vi "Test Broadcast Seen from Process Added After Attaching to Owning Application.vi"(8 "error in (no error)":errorcluster, 11 "Test Case In":refnum<class "Monitor Broadcasts Test.lvclass">) -> (0 "error out":errorcluster, 3 "Test Case Out":refnum<class "Monitor Broadcasts Test.lvclass">)   [LabVIEW 2020, in "Monitor Broadcasts Test.lvclass"]
uses:
  Monitor Broadcasts Test.lvclass
  C:/Program Files (x86)/National Instruments/LabVIEW 2020/vi.lib/Astemes/LUnit/Test Case.lvclass
  source/Broadcast Message Receiver/Broadcast Message Receiver.lvclass
  C:/Git/astemes-triarc-debugger/source/Process/Debug Process.lvclass
  <vilib>/Astemes/Triarc Framework/Application/Application.lvclass
  C:/Program Files (x86)/National Instruments/LabVIEW 2020/vi.lib/Astemes/Triarc Framework/Process/Process.lvclass
  <vilib>/Astemes/Triarc Framework/Process/Process.lvclass
  source/Process/Debug Process.lvclass/Debug Process.ctl
  source/Broadcast Message Receiver/Broadcast Message Receiver.lvclass/Broadcast Message Receiver.ctl
  <vilib>/Astemes/Triarc Framework/Process/Process.lvclass/Process.ctl
  <vilib>/Astemes/Triarc Framework/Application/Application.lvclass/Application.ctl
  <vilib>/Astemes/LUnit/Test Case.lvclass/Test Case.ctl
  b8133177-6539-48d7-afde-5fbce34c741b.vi
  b0973c52-cbc2-441f-a849-3f0b3eb3c153.vi
  01074fa8-ee8a-411d-bc8b-fc92c4f90959.vi
  source/Process/Public/Lifecycle/Get Lifecycle State.vi
  source/Process/Protected/Messaging/Enqueue Message.vi
  <vilib>/Astemes/Triarc Framework/Application/Private/Add Process to Map.vi
  <vilib>/Astemes/Triarc Framework/Application/Private/Throw Error If Process Already in App.vi
  <vilib>/Astemes/Triarc Framework/Process/Protected/Messaging/Send Message.vi
  <vilib>/Astemes/Triarc Framework/Process/Public/Lifecycle/Get Lifecycle State.vi
  <vilib>/Astemes/Triarc Framework/Process/Protected/SubVIs/Set Context.vi
  source/Process/Private/SubVIs/Wait for finish.vi
  source/Process/Private/SubVIs/Set Lifecycle State.vi
  <vilib>/Astemes/Triarc Framework/Process/Private/SubVIs/Wait for finish.vi
  <vilib>/Astemes/Triarc Framework/Process/Private/SubVIs/Set Lifecycle State.vi
  <vilib>/Astemes/LUnit/Palette/Pass.vi
  <vilib>/Astemes/LUnit/Palette/Fail.vi
  <vilib>/Astemes/LUnit/Compare Variants.vi
  <vilib>/Astemes/LUnit/Describe Comparison.vi
  <vilib>/Astemes/LUnit/Set Assertion Type.vi
  <vilib>/Utility/error.llb/Clear Errors.vi
  <vilib>/Astemes/Triarc Framework/Application/Public/Get Process.vi
  <vilib>/Astemes/Triarc Framework/Process/Private/SubVIs/Handle Debug Data.vi
  <vilib>/Astemes/Triarc Framework/Process/Public/Lifecycle/Leave Process Loop.vi
  <vilib>/Astemes/LUnit/Add test result.vi
  <vilib>/Astemes/LUnit/Variant to string.vi
  <vilib>/Astemes/Triarc Framework/Application/Private/Retrieve Process from App.vi
  <vilib>/Astemes/Triarc Framework/Application/Private/Parse Process Name.vi
  <vilib>/Astemes/Triarc Framework/Application/Private/Get Process from Map.vi
  <vilib>/Astemes/Triarc Framework/Logging/Log Debug.vi
  <vilib>/AdvancedString/1D String Array to Delimited String.vi
  <vilib>/Utility/High Resolution Relative Seconds.vi
  <vilib>/Astemes/LUnit/LUnit Record Assertion Result.vi
  <vilib>/Astemes/Triarc Framework/Process/Protected/Messaging/Request Message.vi
  <vilib>/AdvancedString/Delimited String to 1D String Array.vi
  <vilib>/Astemes/LUnit/LUnit Aggregate Assertion Results.vi
  <vilib>/Astemes/Triarc Framework/Process/Private/SubVIs/Enqueue Request Message.vi
  <vilib>/Astemes/LUnit/Method Result/LUnit Merge Status.vi
  <vilib>/Astemes/LUnit/LUnit Concatenate result strings.vi
  source/Mock Data Listener/Mock Data Listener.lvclass
  C:/Git/astemes-triarc-debugger/source/Debug Data Event/Debug Data Listener.lvclass
  <vilib>/Utility/error.llb/Error Cluster From Error Code.vi
  <vilib>/Astemes/Triarc Framework/Process/Public/Read Name.vi
  <vilib>/Astemes/Triarc Framework/Process/Private/SubVIs/Wait for Response Message.vi
  <vilib>/Utility/Data Type/Get Type Information.vi
  <vilib>/Utility/LVClass/Get LV Class Name.vi
  source/Process/Debug Process.lvclass
panel:
  out "x+1":i32
  out "Count":i32
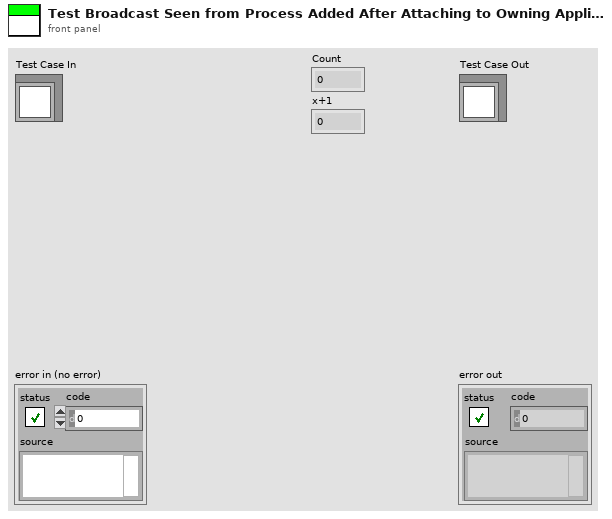
[diagram p1: front panel]
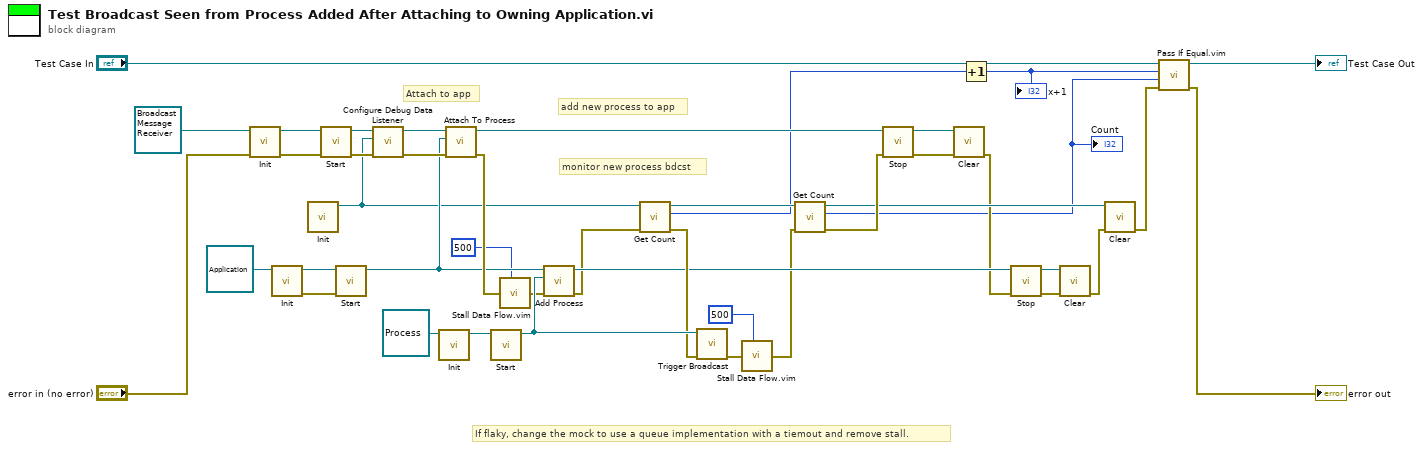
[diagram p0: block diagram]
diagram:
  # "If flaky, change the mock to use a queue implementation with a tiemout and remove stall."
  # "monitor new process bdcst"
  # "add new process to app"
  # "Attach to app"
  n1 = call-dynamic "Init.vi"("error in (no error)"="error in (no error)", "Process In"=refnum<class "Broadcast Message Receiver.lvclass"> refnum ("Broadcast Message Receiver.lvclass")) -> ("error out"=w37:errorcluster, "Process Out"=w38:refnum<class "Broadcast Message Receiver.lvclass">)  [unwired: 8 in]
  n2 = call-dynamic "Init.vi"("Process In"=refnum<class "Application.lvclass"> refnum ("Application In")) -> ("error out"=w25:errorcluster, "Process Out"=w26:refnum<class "Application.lvclass">)  [unwired: 9 in]
  n3 = call "Init.vi"() -> ("Mock Data Listener Out"=w22:refnum<class "Mock Data Listener.lvclass">)  [unwired: 10 in, 1 out]
  n4 = call <vilib>:"Start.vi"("error in (no error)"=w37, "Process In"=w38) -> ("error out"=w35:errorcluster, "Process Out"=w36:refnum<class "Broadcast Message Receiver.lvclass">)  [unwired: 7 in, 1 out]
  n5 = call <vilib>:"Start.vi"("error in (no error)"=w25, "Process In"=w26) -> ("Process Out"=w23:refnum<class "Application.lvclass">)  [unwired: 7 in, 2 out]
  n6 = call "Configure Debug Data Listener.vi"("error in (no error)"=w35, "Debug Data Listener"=w22, "Debug Message Receiver In"=w36) -> ("error out"=w32:errorcluster, "Debug Message Receiver Out"=w34:refnum<class "Broadcast Message Receiver.lvclass">)  [unwired: 7 in]
  n7 = call-dynamic "Init.vi"("Process In"=refnum<class "Process.lvclass"> refnum) -> ("Process Out"=w28:refnum<class "Process.lvclass">)  [unwired: 9 in, 1 out]
  n8 = call "Attach To Process.vi"("error in (no error)"=w32, "Process In"=w23, "Broadcast Message Receiver In"=w34) -> ("error out"=w24:errorcluster, "Broadcast Message Receiver Out"=w33:refnum<class "Broadcast Message Receiver.lvclass">)  [unwired: 7 in]
  n9 = call <vilib>:"Start.vi"("Process In"=w28) -> ("Process Out"=w19:refnum<class "Process.lvclass">)  [unwired: 8 in, 2 out]
  n10 = call "Stall Data Flow.vim"("value in"=w24, "milliseconds to wait"=u32 500) -> ("value out"=w4:errorcluster)  [unwired: 1 out]
  n11 = call <vilib>:"Add Process.vi"("error in (no error)"=w4, "Process"=w19, "Application In"=w23) -> ("error out"=w5:errorcluster, "Application Out"=w13:refnum<class "Application.lvclass">)  [unwired: 7 in]
  n12 = call "Get Count.vi"("error in (no error)"=w5, "Mock Data Listener In"=w22) -> ("error out"=w18:errorcluster, "Count"=w8:i32, "Mock Data Listener Out"=w21:refnum<class "Mock Data Listener.lvclass">)  [unwired: 7 in]
  n13 = call <vilib>:"Trigger Broadcast.vi"("error in (no error)"=w18, "Process in"=w19) -> ("error out"=w17:errorcluster)  [unwired: 8 in, 1 out]
  n14 = call "Stall Data Flow.vim"("value in"=w17, "milliseconds to wait"=u32 500) -> ("value out"=w2:errorcluster)  [unwired: 1 out]
  n15 = call "Get Count.vi"("error in (no error)"=w2, "Mock Data Listener In"=w21) -> ("error out"=w20:errorcluster, "Count"=w6:i32, "Mock Data Listener Out"=w12:refnum<class "Mock Data Listener.lvclass">)  [unwired: 7 in]
  "Count" <- w6
  n16 = call <vilib>:"Stop.vi"("error in (no error)"=w20, "Process In"=w33) -> ("error out"=w30:errorcluster, "Process Out"=w31:refnum<class "Broadcast Message Receiver.lvclass">)  [unwired: 7 in, 1 out]
  n17 = call-dynamic "Clear.vi"("error in (no error)"=w30, "Process In"=w31) -> ("error out"=w10:errorcluster)  [unwired: 9 in]
  n18 = Increment(x=w8) -> (x+1=w7:i32)
  "x+1" <- w7
  n19 = call <vilib>:"Stop.vi"("error in (no error)"=w10, "Process In"=w13) -> ("error out"=w14:errorcluster, "Process Out"=w15:refnum<class "Application.lvclass">)  [unwired: 7 in, 1 out]
  n20 = call-dynamic "Clear.vi"("error in (no error)"=w14, "Application In"=w15) -> ("error out"=w11:errorcluster)  [unwired: 9 in]
  n21 = call "Clear.vi"("error in (no error)"=w11, "Mock Data Listener in"=w12) -> ("error out"=w9:errorcluster)  [unwired: 9 in]
  n22 = call "Pass If Equal.vim"("error in (no error)"=w9, "Actual"=w6, "Expected"=w7, "LUnit Test Case In"="Test Case In") -> ("error out"=→"error out":errorcluster, "LUnit Test Case Out"=→"Test Case Out":refnum<class "Monitor Broadcasts Test.lvclass">)  [unwired: 6 in]
